vi "ActionVIOnSave.vi"(8 "error in (no error)":errorcluster, 11 "Device Item Ref in":T1 format="%.0x") -> (0 "error out":errorcluster, 3 "Device Item Ref out":T1 format="%.0x")   [LabVIEW 2019, in "UDP-Custom-Device System Explorer.lvlib"]
uses:
  UDP-Custom-Device System Explorer.lvlib
  <vilib>/NI VeriStand/Custom Device API/Custom Device Item Ref.ctl
  Property Accessors/Main Accessors.lvlib
  <vilib>/NI VeriStand/Custom Device API/Custom Device API.lvlib
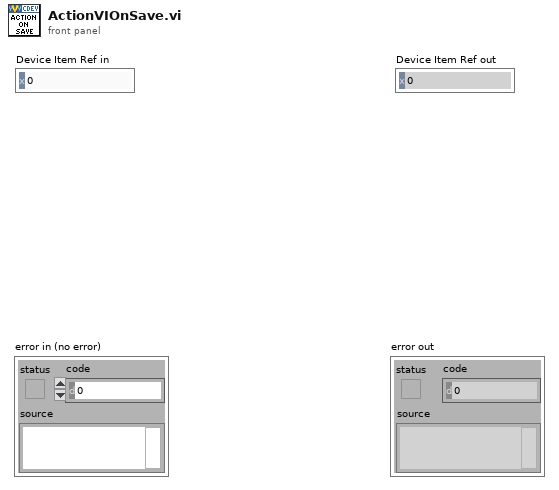
[diagram p1: front panel]
types:
  T1 = typedef "Custom Device API.lvlib/Custom Device Item Ref.ctl" = u64
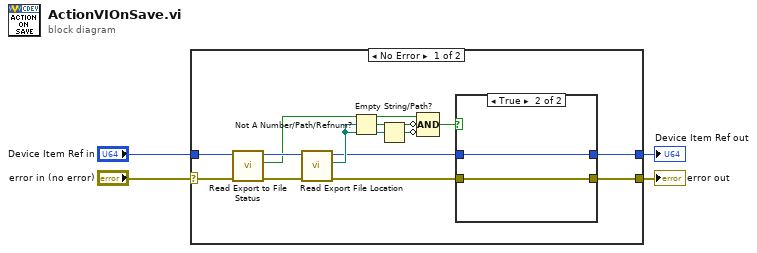
[diagram p0: block diagram]
diagram:
  n1 = case shown="No Error" "error in (no error)" {
    selector: "error in (no error)" -> [w16 w23]
    tunnel: [w15 w23] -> w3
    tunnel: "Device Item Ref in" -> [w17 w22]
    tunnel: [w14 w22] -> w1
    frame No Error {
      n2 = call "Read Export to File Status.vi"("error in (no error)"=w16, "Node Ptr"=w17) -> ("error out"=w12:errorcluster, "Export to File Status"=w11:bool, "Node Ptr out"=w13:T1)  [unwired: 7 in]
      n3 = call "Read Export File Location.vi"("error in (no error)"=w12, "Node Ptr"=w13) -> ("error out"=w6:errorcluster, "Export File Location"=w9:path, "Node Ptr out"=w7:T1)  [unwired: 7 in]
      n4 = Not A Number/Path/Refnum?(number/path/refnum=w9) -> (NaN/Path/Refnum?=w10:bool)
      n5 = Empty String/Path?(string/path=w9) -> (empty?=w8:bool)
      n6 = Compound Arithmetic op=AND(w11, invert w10, invert w8) -> (w5:bool)
      n7 = case shown="True" w5 {
        tunnel: w7 -> [w19 w21]
        tunnel: w6 -> [w18 w20]
        tunnel: [w18 w20] -> w15
        tunnel: [w19 w21] -> w14
        frame False {
        }
        frame True {
        }
      }
    }
    frame Error {
    }
  }
  "error out" <- w3
  "Device Item Ref out" <- w1
